vi "Acknowledgement User Event.vi"(0 "ACK":T1, 11 "Error in":errorcluster, 13 "Operations":T2) -> (4 "ACK Event":refnum<user-event>, 15 "Error out":errorcluster)   [LabVIEW 2020, in "Data Communication Receiver.lvlib"]
doc: "This is a User event LV2 which is basically used to trigger an acknowledgement to the transmitter which is sending data to this receiver."
uses:
  Data Communication Receiver.lvlib
  Typedefs/User event Operations.ctl
  Typedefs/User Event Stop Data.ctl
  Transmitter/Data Communication Transmitter.lvlib
panel:
  # "ACKNOWLEDGEMENT EVENT"
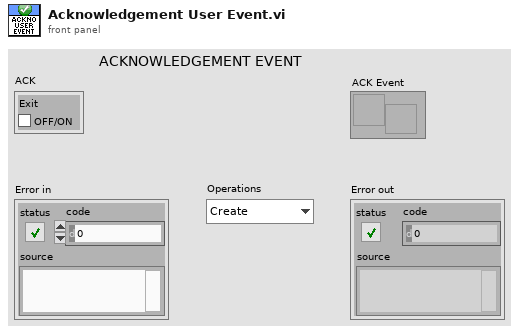
[diagram p1: front panel]
types:
  T1 = typedef "Data Communication Receiver.lvlib/User Event Stop Data.ctl" = cluster{"Exit":bool}
  T2 = typedef "Data Communication Transmitter.lvlib/User event Operations.ctl" = enum16{"Create", "Generate", "Get Ref", "destroy"}
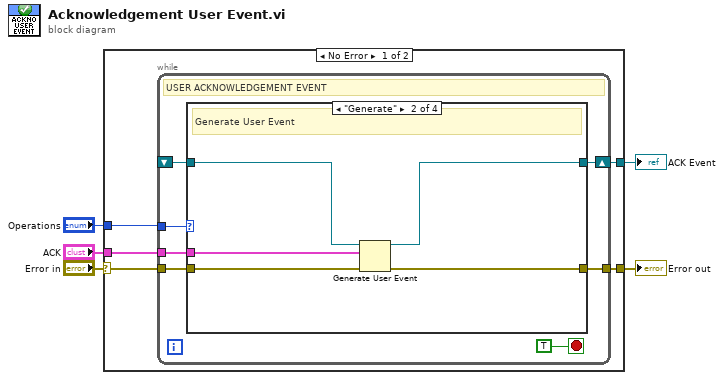
[diagram p0: block diagram]
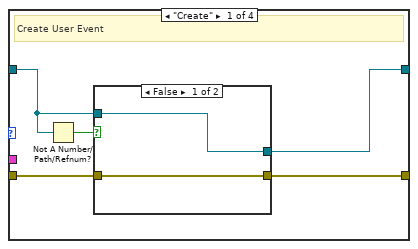
[diagram p2: hidden frame]
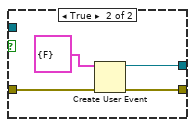
[diagram p3: hidden frame]
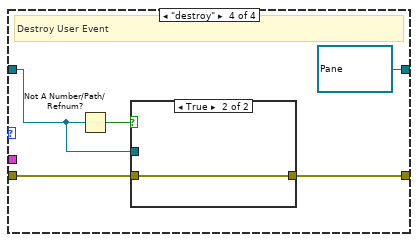
[diagram p5: hidden frame]
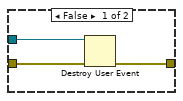
[diagram p6: hidden frame]
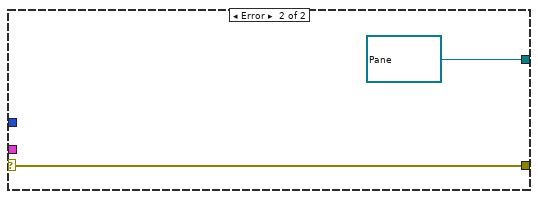
[diagram p7: hidden frame]
diagram:
  n1 = case shown="No Error" "Error in" {
    selector: "Error in" -> [w10 w46]
    tunnel: [w9 w46] -> w4
    tunnel: "Operations" -> [w8 _]
    tunnel: "ACK" -> [w7 _]
    tunnel: [w6 refnum<user-event> refnum ("Stop")] -> w1
    frame No Error {
      n2 = while {
        tunnel: w8 -> [w16]
        tunnel: w10 -> [w15]
        tunnel: [w14] -> w9
        shift-right: [w13] -> w6
        shift-left: _ -> [w12]
        tunnel: w7 -> [w11]
        stop <- TRUE stop-if-true
        # "USER ACKNOWLEDGEMENT EVENT"
        n3 = case shown="\"Generate\"" w16 {
          tunnel: w15 -> [w22 w33 w35 w40]
          tunnel: [w21 w32 w35 w39] -> w14
          tunnel: [w20 w30 w34 refnum<user-event> refnum ("Stop")] -> w13
          tunnel: w12 -> [w19 w31 w34 w37]
          tunnel: w11 -> [_ w29 _ _]
          frame "Create" {
            # "Create User Event"
            n4 = Not A Number/Path/Refnum?(number/path/refnum=w19) -> (NaN/Path/Refnum?=w18:bool)
            n5 = case shown="False" w18 {
              tunnel: w22 -> [w24 w28]
              tunnel: [w24 w27] -> w21
              tunnel: [w23 w26] -> w20
              tunnel: w19 -> [w23 _]
              frame False {
              }
              frame True {
                n6 = Create User Event(user event datatype=T1 {"Exit"=FALSE} ("ACK"), error in=w28) -> (user event=w26:refnum<user-event>, error out=w27:errorcluster)
              }
            }
          }
          frame "Generate" {
            # "Generate User Event"
            n7 = Generate User Event(user event=w31, event data cluster=w29, error in=w33) -> (user event out=w30:refnum<user-event>, error out=w32:errorcluster)  [unwired: 1 in]
          }
          frame "Get Ref" {
            # "Get User Event Reference"
          }
          frame "destroy" {
            # "Destroy User Event"
            n8 = Not A Number/Path/Refnum?(number/path/refnum=w37) -> (NaN/Path/Refnum?=w38:bool)
            n9 = case shown="True" w38 {
              tunnel: w40 -> [w43 w44]
              tunnel: [w42 w44] -> w39
              tunnel: w37 -> [w41 _]
              frame False {
                n10 = Destroy User Event(user event=w41, error in=w43) -> (error out=w42:errorcluster)
              }
              frame True {
              }
            }
          }
        }
      }
    }
    frame Error {
    }
  }
  "Error out" <- w4
  "ACK Event" <- w1
